vi "ErrorLogDialog.vi"() -> (3 "Cancelled?":bool)   [LabVIEW 2018]
doc: "*-----------------------------------------------------\n* Author: SWatts\n*\n* VI Description: Error Log Viewer\n* \n*\n* Error handling: All errors passed out\n*\n* Pre-condition: \n*\n* Post-condition: None\n*\n* Revision History:\n*\n* Rev Date Author Description \n* 01 30/04/2014 SWatts First issue\n*\n*-----------------------------------------------------"
uses:
  ErrordBCommand.ctl
  Controls/DisplayQCommand.ctl
  Controls/DisplayMessage.ctl
panel:
  in  "Error History":i32(listbox)
  in  "Clear Alarm":bool
  in  "OK":bool
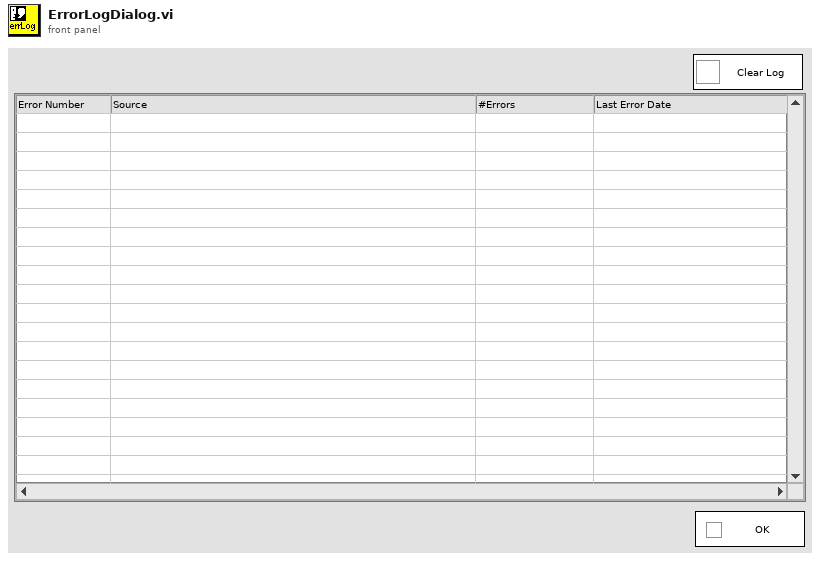
[diagram p1: front panel]
types:
  T1 = typedef "ErrordBCommand.ctl" = enum16{"No Command - Error", "Get All Errors", "Get #Errors", "Clear Error Log", "Insert New Error", "Update Existing Error"}
  T2 = typedef "DisplayMessage.ctl" = enum16{"No Message - Ignore", "Display Message", "Set Tab", "Set Status", "Add Error Message", "Clear Error History", "Generate Error", "Set Idling Display", "Set Running Display", "Stop"}
  T3 = typedef "DisplayQCommand.ctl" = enum16{"No Command - Error", "Initialise", "Get Q Reference", "Add Item to Bottom", "Add Item to Top", "Flush Q", "Dequeue", "Peek Next Element", "Close"}
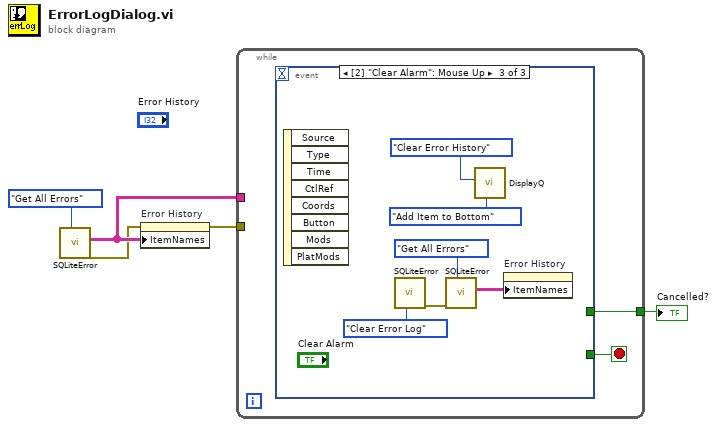
[diagram p0: block diagram]
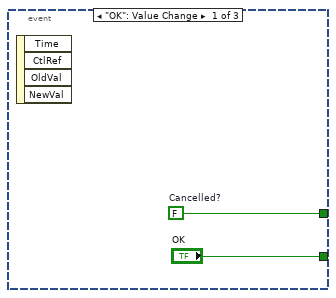
[diagram p2: hidden frame]
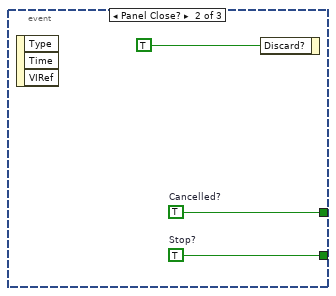
[diagram p3: hidden frame]
diagram:
  n1 = call "SQLiteError.vi"("ConfigCommand"=ErrordBCommand."Get All Errors") -> ("error out"=w2:errorcluster, "All Errors"=w3:string[][])  [unwired: 5 in, 1 out]
  n2 = property on="Error History" class="MCListbox (strict)"(error in=w2, "ItemNames"=w3) -> (error out=w1:errorcluster)  [unwired: 1 in, 1 out]
  n3 = while {
    tunnel: [w6] -> w5
    tunnel: w3 -> [_]
    tunnel: w1 -> [_]
    stop <- w7 stop-if-true
    n4 = event shown="[2] \"Clear Alarm\": Mouse Up" {
      selector: _ -> [_ _ _]
      dyn-events: _ -> [_ _ _]
      timeout: _ -> [_ _ _]
      tunnel: ["OK" w11 _] -> w7
      tunnel: [w9 w10 _] -> w6
      event "OK": Value Change {
        w9 = FALSE  # Cancelled?
        n5 = event-data() -> ()  [unwired: 1 in, 4 out]
      }
      event Panel Close? {
        w10 = TRUE  # Cancelled?
        w11 = TRUE  # Stop?
        n6 = event-data() -> ()  [unwired: 1 in, 3 out]
        n7 = event-data("Discard?"=TRUE) -> ()  [unwired: 1 in, 1 out]
      }
      event "Clear Alarm": Mouse Up {
        n8 = event-data() -> ()  [unwired: 1 in, 8 out]
        n9 = call "SQLiteError.vi"("ConfigCommand"=ErrordBCommand."Clear Error Log") -> ("error out"=w17:errorcluster)  [unwired: 5 in, 2 out]
        n10 = call "SQLiteError.vi"("ConfigCommand"=ErrordBCommand."Get All Errors", "error in (no error)"=w17) -> ("All Errors"=w15:string[][])  [unwired: 4 in, 2 out]
        n11 = call "DisplayQ.vi"("command"=DisplayQCommand."Add Item to Bottom", "DisplayMessage"=DisplayMessage."Clear Error History") -> ()  [unwired: 3 in, 4 out]
        n12 = property on="Error History" class="MCListbox (strict)"("ItemNames"=w15) -> ()  [unwired: 2 in, 2 out]
      }
    }
  }
  "Cancelled?" <- w5
